vi "fetch_and_translate_trigger.vi"(8 "error in (no error)":errorcluster, 11 "StimulatorDL090503Scaffold in":refnum<class "StimulatorDL090503Scaffold.lvclass">) -> (0 "error out":errorcluster, 1 "sender TLC type":T1=enum."ImagingMode", 2 "statechart trigger":T2, 3 "StimulatorDL090503Scaffold out":refnum<class "StimulatorDL090503Scaffold.lvclass">)   [LabVIEW 2010, in "StimulatorDL090503Scaffold.lvclass"]
uses:
  StimulatorDL090503Scaffold.lvclass
  internal_trigger_enum.ctl
  common/enumerations/top-level_component_type_enum.ctl
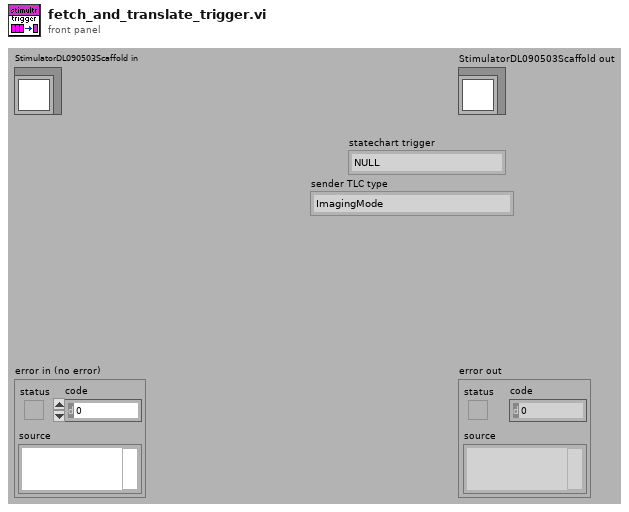
[diagram p1: front panel]
types:
  T1 = typedef "top-level_component_type_enum.ctl" = enum16{"undefined", "ImagingMode", "ScanHead", "DAQ", "ImageAssembler", "Display", "DataCollection", "Analyser", "Stimulator", "ExperimentController", "Instrument", "Stage"}
  T2 = typedef "StimulatorDL090503Scaffold.lvclass/internal_trigger_enum.ctl" = enum16{"NULL", "initialise", "terminate", "start sweep", "stop sweep", "start stimulation", "stop stimulation"}
  T3 = typedef "GenericToplevelComponent.lvclass/common_trigger_enum.ctl" = enum16{"NULL", "initialise", "terminate", "fetch command", "fetch data", "attach observer", "register as observer", "detach observer", "acknowledge", "start", "stop", "sweep started", "sweep finished", "experiment started", "experiment stopped"}
  T4 = typedef "trigger_type_enum.ctl" = enum8{"external", "internal", "common"}
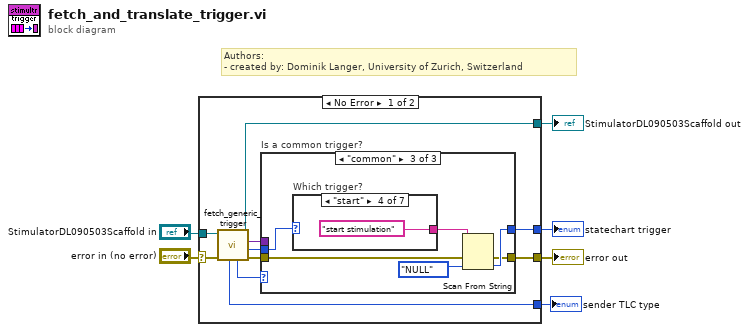
[diagram p0: block diagram]
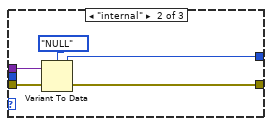
[diagram p3: hidden frame]
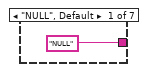
[diagram p4: hidden frame]
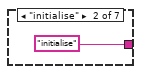
[diagram p5: hidden frame]
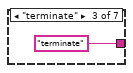
[diagram p6: hidden frame]
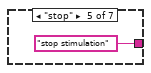
[diagram p7: hidden frame]
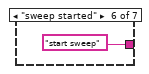
[diagram p8: hidden frame]
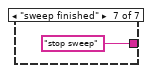
[diagram p9: hidden frame]
diagram:
  # "Authors: \n- created by: Dominik Langer, University of Zurich, Switzerland"
  n1 = case shown="No Error" "error in (no error)" {
    selector: "error in (no error)" -> [w15 w37]
    tunnel: [w10 w37] -> w5
    tunnel: [w13 w36] -> w3
    tunnel: "StimulatorDL090503Scaffold in" -> [w14 w36]
    tunnel: [w16 _] -> w1
    tunnel: [w7 _] -> w2
    frame No Error {
      n2 = call-dynamic "fetch_generic_trigger.vi"("error in (no error)"=w15, "GenericToplevelComponent in"=w14) -> ("error out"=w11:errorcluster, "common trigger"=w8:T3, "trigger"=w12:variant, "GenericToplevelComponent out"=w13:refnum<class "StimulatorDL090503Scaffold.lvclass">, "trigger type"=w9:T4, "sender TLC type"=w7:T1)  [unwired: 3 in, 1 out]
      n3 = case "Is a common trigger?" shown="\"common\"" w9 {
        tunnel: [_ w19 w25] -> w16
        tunnel: w12 -> [_ w22 _]
        tunnel: w11 -> [w17 w21 w24]
        tunnel: [w17 w20 w23] -> w10
        tunnel: w8 -> [_ _ w28]
        frame "external", Default {
          # "GenericStimulator does not provide external triggers."
        }
        frame "internal" {
          n4 = Variant To Data(error in=w21, Variant=w22, type=internal_trigger_enum."NULL" ("statechart trigger")) -> (error out=w20:errorcluster, data=w19:T2)
        }
        frame "common" {
          n5 = case "Which trigger?" shown="\"start\"" w28 {
            tunnel: ["NULL" "initialise" "terminate" "start stimulation" "stop stimulation" "start sweep" "stop sweep"] -> w27
            frame "NULL", Default {
            }
            frame "initialise" {
            }
            frame "terminate" {
            }
            frame "start" {
            }
            frame "stop" {
            }
            frame "sweep started" {
            }
            frame "sweep finished" {
            }
          }
          n6 = Scan From String(input string=w27, error in=w24, default 1=internal_trigger_enum."NULL" ("statechart trigger")) -> (error out=w23:errorcluster, output 1=w25:T2)  [unwired: 2 in, 2 out]
        }
      }
    }
    frame Error {
    }
  }
  "error out" <- w5
  "StimulatorDL090503Scaffold out" <- w3
  "statechart trigger" <- w1
  "sender TLC type" <- w2
